vi "Start Drag.vi"(8 "error in (no error)":errorcluster, 9 "Snap size":dbl=1.0, 11 "FSM in":refnum<class "FSM.Node.lvclass">) -> (0 "error out":errorcluster, 3 "FSM out":refnum<class "FSM.Node.lvclass">)   [LabVIEW 2015, in "FSM.Node.lvclass"]
uses:
  FSM.Node.lvclass
  FSM.Node.lvclass/FSM.Node.ctl
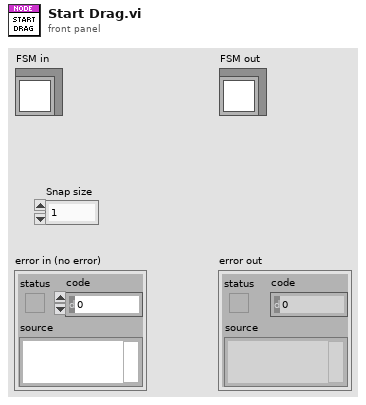
[diagram p1: front panel]
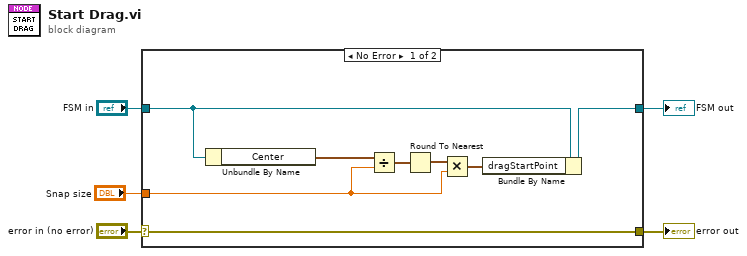
[diagram p0: block diagram]
diagram:
  n1 = case shown="No Error" "error in (no error)" {
    selector: "error in (no error)" -> [w13 w15]
    tunnel: [w13 w15] -> w4
    tunnel: [w7 w14] -> w2
    tunnel: "FSM in" -> [w12 w14]
    tunnel: "Snap size" -> [w8 _]
    frame No Error {
      n2 = Unbundle By Name(w12) -> ("Center"=w11:cluster{"X":dbl, "Y":dbl})
      n3 = Divide(x=w11, y=w8) -> (x/y=w10:cluster{"X":dbl, "Y":dbl})
      n4 = Round To Nearest(number=w10) -> (nearest integer value=w9:cluster{"X":dbl, "Y":dbl})
      n5 = Multiply(x=w9, y=w8) -> (x*y=w6:cluster{"X":dbl, "Y":dbl})
      n6 = Bundle By Name(cluster=w12, "dragStartPoint"=w6) -> (w7:refnum<class "FSM.Node.lvclass">)
    }
    frame Error {
    }
  }
  "error out" <- w4
  "FSM out" <- w2
